vi "练习1.2-波形测量.vi"() -> ()   [LabVIEW 2021]
panel:
  out "f 2":dbl
  out "f 1":dbl
  in  "stop":bool
  out "Waveform Graph":dynamicdata(graph)
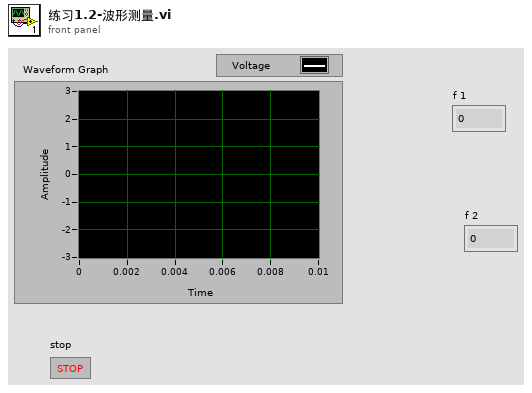
[diagram p1: front panel]
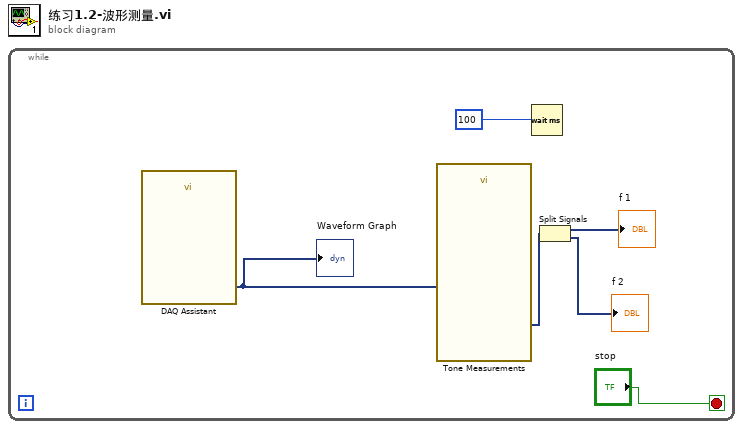
[diagram p0: block diagram]
diagram:
  n1 = while {
    stop <- "stop" stop-if-true
    n2 = call "DAQ Assistant"() -> ("data"=w4:dynamicdata)  [unwired: 17 in, 2 out]
    "Waveform Graph" <- w4
    n3 = call "Tone Measurements"("Signals"=w4) -> ("Frequency"=w3:dynamicdata)  [unwired: 7 in, 3 out]
    n4 = Wait (ms)(milliseconds to wait=100) -> ()  [unwired: 1 out]
    n5 = Split Signals(w3) -> (→"f 1":dynamicdata, →"f 2":dynamicdata)  [unwired: 2 in]
  }
